vi "Lesson 3 - Exercise 3.1.2 - Cos Sin Orthogonality.vi"() -> ()   [LabVIEW 2015]
uses:
  <vilib>/Analysis/NI_AALBase.lvlib
panel:
  in  "A":dbl=3.0
  in  "B":dbl=3.0
  in  "stop":bool
  out "2*Avg( [A*Sin+B*Cos] * Sin )":dbl=2.9999999999999996 format="%.2f"
  out "1 * Sin(f)":dbl[](graph)=[0.0, 0.049067674327418015, 0.0980171403295606, 0.14673047445536175, 0.19509032201612828, 0.2429801799032639, 0.2902846772544624, 0.33688985339222005, 0.3826834323650898, 0.4275550934302821, 0.47139673682599764, 0.5141027441932218, 0.5555702330196022, 0.5956993044924334, 0.6343932841636455, 0.6715589548470184, 0.7071067811865475, 0.7409511253549591, 0.7730104533627369, 0.8032075314806449, 0.8314696123025451, 0.8577286100002721, 0.8819212643483549, 0.9039892931234433, 0.9238795325112866, 0.9415440651830208, 0.9569403357322087, 0.970031253194544, 0.9807852804032303, 0.9891765099647809, 0.9951847266721968, 0.9987954562051723, 0.9999999999999999, 0.9987954562051723, 0.9951847266721968, 0.9891765099647809, 0.9807852804032304, 0.970031253194544, 0.9569403357322088, 0.9415440651830208, 0.9238795325112867, 0.9039892931234433, 0.881921264348355, 0.8577286100002721, 0.8314696123025452, 0.8032075314806449, 0.773010453362737, 0.7409511253549591, 0.7071067811865476, 0.6715589548470184, 0.6343932841636456, 0.5956993044924334, 0.5555702330196023, 0.5141027441932218, 0.4713967368259977, 0.42755509343028214, 0.38268343236508984, 0.3368898533922201, 0.29028467725446244, 0.24298017990326393, 0.19509032201612836, 0.14673047445536178, 0.0980171403295607, 0.04906767432741803, 1.0034968732711147e-16, -0.04906767432741801, -0.0980171403295605, -0.14673047445536175, -0.19509032201612816, -0.2429801799032639, -0.2902846772544623, -0.33688985339222005, -0.38268343236508967, -0.4275550934302821, -0.47139673682599753, -0.5141027441932218, -0.5555702330196021, -0.5956993044924334, -0.6343932841636454, -0.6715589548470184, -0.7071067811865475, -0.7409511253549591, -0.7730104533627369, -0.8032075314806449, -0.8314696123025451, -0.8577286100002721, -0.8819212643483549, -0.9039892931234433, -0.9238795325112866, -0.9415440651830208, -0.9569403357322087, -0.970031253194544, -0.9807852804032303, -0.9891765099647809, -0.9951847266721968, -0.9987954562051723, -0.9999999999999999, -0.9987954562051723, -0.9951847266721968, -0.9891765099647809, -0.9807852804032304, -0.970031253194544, -0.9569403357322088, -0.9415440651830208, -0.9238795325112867, -0.9039892931234433, -0.881921264348355, -0.8577286100002721, -0.8314696123025452, -0.8032075314806449, -0.773010453362737, -0.7409511253549591, -0.7071067811865476, -0.6715589548470184, -0.6343932841636456, -0.5956993044924334, -0.5555702330196023, -0.5141027441932218, -0.4713967368259977, -0.42755509343028214, -0.38268343236508984, -0.3368898533922201, -0.29028467725446244, -0.24298017990326395, -0.19509032201612836, -0.1467304744553618, -0.0980171403295607, -0.049067674327418064]
  out "B * Cos(f)":dbl[](graph)=[3.0, 2.996386368615517, 2.9855541800165906, 2.967529529894343, 2.9423558412096913, 2.910093759583632, 2.8708210071966267, 2.824632195549062, 2.7716385975338604, 2.71196787937033, 2.6457637930450653, 2.573185830000816, 2.494408836907636, 2.4096225944419345, 2.319031360088211, 2.222853376064877, 2.121320343559643, 2.0146768645410553, 1.9031798524909367, 1.7870979134773002, 1.6667106990588068, 1.5423082325796653, 1.414190210477993, 1.2826652802908465, 1.1480502970952695, 1.0106695601766604, 0.8708540317633873, 0.728940539709792, 0.5852709660483849, 0.4401914233660856, 0.29405142098868187, 0.14720302298225438, 3.472157457384828e-17, -0.1472030229822537, -0.2940514209886818, -0.4401914233660849, -0.5852709660483848, -0.7289405397097913, -0.8708540317633872, -1.0106695601766598, -1.1480502970952693, -1.2826652802908458, -1.4141902104779929, -1.5423082325796647, -1.6667106990588065, -1.7870979134772995, -1.9031798524909365, -2.014676864541055, -2.1213203435596424, -2.2228533760648768, -2.3190313600882106, -2.409622594441934, -2.4944088369076356, -2.5731858300008157, -2.645763793045065, -2.7119678793703295, -2.77163859753386, -2.8246321955490616, -2.8708210071966263, -2.9100937595836314, -2.942355841209691, -2.9675295298943425, -2.98555418001659, -2.996386368615517, -2.9999999999999996, -2.996386368615517, -2.98555418001659, -2.967529529894343, -2.942355841209691, -2.9100937595836323, -2.8708210071966263, -2.8246321955490625, -2.77163859753386, -2.7119678793703303, -2.645763793045065, -2.5731858300008166, -2.4944088369076356, -2.409622594441935, -2.3190313600882106, -2.2228533760648777, -2.1213203435596424, -2.0146768645410558, -1.9031798524909365, -1.7870979134773006, -1.6667106990588068, -1.5423082325796658, -1.414190210477993, -1.282665280290847, -1.1480502970952695, -1.0106695601766609, -0.8708540317633874, -0.7289405397097924, -0.5852709660483851, -0.440191423366086, -0.2940514209886822, -0.1472030229822548, -4.4368263403538055e-16, 0.1472030229822533, 0.2940514209886813, 0.4401914233660845, 0.5852709660483842, 0.728940539709791, 0.8708540317633865, 1.0106695601766595, 1.1480502970952686, 1.2826652802908458, 1.4141902104779922, 1.5423082325796647, 1.6667106990588059, 1.7870979134772995, 1.9031798524909356, 2.014676864541055, 2.1213203435596415, 2.222853376064877, 2.3190313600882098, 2.409622594441935, 2.4944088369076347, 2.5731858300008166, 2.645763793045064, 2.7119678793703303, 2.771638597533859, 2.8246321955490625, 2.8708210071966254, 2.9100937595836323, 2.94235584120969, 2.9675295298943434, 2.9855541800165892, 2.996386368615518]
  out "A * Sin(f)":dbl[](graph)=[0.0, 0.14720302298225404, 0.2940514209886818, 0.44019142336608524, 0.5852709660483848, 0.7289405397097917, 0.8708540317633872, 1.0106695601766602, 1.1480502970952693, 1.2826652802908463, 1.4141902104779929, 1.542308232579665, 1.6667106990588065, 1.7870979134773, 1.9031798524909365, 2.0146768645410553, 2.1213203435596424, 2.222853376064877, 2.3190313600882106, 2.4096225944419345, 2.4944088369076356, 2.573185830000816, 2.645763793045065, 2.71196787937033, 2.77163859753386, 2.824632195549062, 2.8708210071966263, 2.910093759583632, 2.942355841209691, 2.967529529894343, 2.98555418001659, 2.996386368615517, 2.9999999999999996, 2.996386368615517, 2.98555418001659, 2.967529529894343, 2.942355841209691, 2.910093759583632, 2.8708210071966263, 2.824632195549062, 2.77163859753386, 2.71196787937033, 2.645763793045065, 2.573185830000816, 2.4944088369076356, 2.4096225944419345, 2.3190313600882106, 2.222853376064877, 2.1213203435596424, 2.0146768645410553, 1.9031798524909365, 1.7870979134773002, 1.6667106990588068, 1.5423082325796653, 1.414190210477993, 1.2826652802908465, 1.1480502970952695, 1.0106695601766604, 0.8708540317633874, 0.728940539709792, 0.5852709660483851, 0.4401914233660856, 0.29405142098868214, 0.14720302298225435, 3.703363570667362e-16, -0.14720302298225374, -0.2940514209886814, -0.44019142336608497, -0.5852709660483844, -0.7289405397097914, -0.8708540317633866, -1.01066956017666, -1.1480502970952688, -1.282665280290846, -1.4141902104779924, -1.5423082325796649, -1.666710699058806, -1.7870979134772997, -1.9031798524909358, -2.014676864541055, -2.121320343559642, -2.2228533760648768, -2.31903136008821, -2.409622594441934, -2.494408836907635, -2.5731858300008157, -2.6457637930450644, -2.7119678793703295, -2.7716385975338595, -2.8246321955490616, -2.870821007196626, -2.9100937595836314, -2.9423558412096904, -2.9675295298943425, -2.9855541800165897, -2.996386368615517, -2.999999999999999, -2.996386368615517, -2.9855541800165897, -2.967529529894343, -2.9423558412096904, -2.9100937595836323, -2.870821007196626, -2.8246321955490625, -2.7716385975338595, -2.7119678793703303, -2.6457637930450644, -2.5731858300008166, -2.494408836907635, -2.409622594441935, -2.3190313600882106, -2.2228533760648777, -2.1213203435596424, -2.0146768645410558, -1.9031798524909365, -1.7870979134773006, -1.6667106990588068, -1.5423082325796658, -1.414190210477993, -1.282665280290847, -1.1480502970952695, -1.0106695601766609, -0.8708540317633874, -0.7289405397097924, -0.5852709660483851, -0.440191423366086, -0.29405142098868225, -0.1472030229822548]
  out "A*Sin + B*Cos":dbl[](graph)=[3.0, 3.143589391597771, 3.2796056010052723, 3.4077209532604282, 3.527626807258076, 3.6390342992934235, 3.7416750389600137, 3.8353017557257223, 3.9196888946291297, 3.994633159661176, 4.059954003523059, 4.115494062580481, 4.161119535966442, 4.196720507919235, 4.222211212579148, 4.237530240605933, 4.242640687119286, 4.237530240605933, 4.222211212579147, 4.196720507919235, 4.161119535966442, 4.115494062580481, 4.059954003523058, 3.994633159661176, 3.9196888946291297, 3.8353017557257223, 3.7416750389600137, 3.639034299293424, 3.5276268072580756, 3.4077209532604287, 3.279605601005272, 3.1435893915977715, 2.9999999999999996, 2.8491833456332634, 2.6915027590279084, 2.527338106528258, 2.357084875161306, 2.1811532198738406, 1.9999669754332392, 1.8139626353724023, 1.6235883004385907, 1.429302599079484, 1.231573582567072, 1.0308775974211515, 0.8276981378488291, 0.622524680964635, 0.4158515075972742, 0.20817651152382233, 0.0, -0.20817651152382144, -0.4158515075972742, -0.6225246809646339, -0.8276981378488288, -1.0308775974211504, -1.2315735825670717, -1.429302599079483, -1.6235883004385905, -1.8139626353724012, -1.9999669754332388, -2.1811532198738393, -2.3570848751613056, -2.5273381065282567, -2.691502759027908, -2.8491833456332625, -2.999999999999999, -3.1435893915977706, -3.2796056010052714, -3.407720953260428, -3.527626807258075, -3.6390342992934235, -3.741675038960013, -3.8353017557257223, -3.919688894629129, -3.994633159661176, -4.059954003523057, -4.115494062580481, -4.161119535966442, -4.196720507919235, -4.222211212579147, -4.237530240605933, -4.242640687119284, -4.237530240605933, -4.222211212579147, -4.196720507919235, -4.161119535966442, -4.115494062580481, -4.059954003523058, -3.994633159661176, -3.919688894629129, -3.8353017557257223, -3.7416750389600133, -3.639034299293424, -3.5276268072580756, -3.4077209532604287, -3.279605601005272, -3.143589391597772, -2.9999999999999996, -2.849183345633264, -2.6915027590279084, -2.5273381065282585, -2.357084875161306, -2.181153219873841, -1.9999669754332392, -1.813962635372403, -1.623588300438591, -1.4293025990794845, -1.2315735825670722, -1.030877597421152, -0.8276981378488293, -0.6225246809646354, -0.41585150759727507, -0.20817651152382277, -8.881784197001252e-16, 0.20817651152382144, 0.4158515075972733, 0.6225246809646343, 0.827698137848828, 1.0308775974211508, 1.2315735825670708, 1.4293025990794834, 1.6235883004385896, 1.8139626353724017, 1.9999669754332379, 2.1811532198738397, 2.3570848751613047, 2.527338106528257, 2.691502759027907, 2.849183345633263]
  out "[A*Sin + B*Cos] * Sin":dbl[](graph)=[0.0, 0.15424862048604557, 0.3214575624193467, 0.5000165122833803, 0.6882058497807045, 0.8842132087164639, 1.0861509310755855, 1.2920742462013628, 1.5, 1.7079257537986372, 1.9138490689244148, 2.115786791283536, 2.311794150219295, 2.49998348771662, 2.6785424375806537, 2.845751379513955, 3.0, 3.1398028005026366, 3.263813403629037, 3.370837519480007, 3.459844447314564, 3.5299770017615293, 3.5805597679832206, 3.6111056062895734, 3.6213203435596424, 3.6111056062895734, 3.5805597679832206, 3.5299770017615293, 3.459844447314564, 3.3708375194800073, 3.263813403629037, 3.139802800502636, 2.999999999999999, 2.8457513795139544, 2.678542437580653, 2.49998348771662, 2.311794150219295, 2.1157867912835364, 1.913849068924414, 1.7079257537986374, 1.4999999999999998, 1.2920742462013632, 1.0861509310755852, 0.8842132087164644, 0.6882058497807045, 0.5000165122833805, 0.3214575624193466, 0.15424862048604576, 0.0, -0.13980280050263583, -0.263813403629038, -0.3708375194800064, -0.45984444731456475, -0.5299770017615287, -0.5805597679832211, -0.6111056062895734, -0.6213203435596425, -0.6111056062895734, -0.5805597679832212, -0.5299770017615288, -0.4598444473145648, -0.37083751948000676, -0.26381340362903827, -0.13980280050263624, -3.010490619813343e-16, 0.1542486204860455, 0.3214575624193463, 0.5000165122833802, 0.688205849780704, 0.8842132087164639, 1.0861509310755848, 1.2920742462013628, 1.4999999999999993, 1.7079257537986372, 1.9138490689244134, 2.115786791283536, 2.3117941502192947, 2.49998348771662, 2.6785424375806524, 2.845751379513955, 2.9999999999999987, 3.1398028005026366, 3.263813403629037, 3.370837519480007, 3.459844447314564, 3.5299770017615293, 3.5805597679832206, 3.6111056062895734, 3.6213203435596415, 3.6111056062895734, 3.58055976798322, 3.5299770017615293, 3.459844447314564, 3.3708375194800073, 3.263813403629037, 3.1398028005026366, 2.999999999999999, 2.845751379513955, 2.678542437580653, 2.4999834877166203, 2.311794150219295, 2.115786791283537, 1.913849068924414, 1.707925753798638, 1.5, 1.2920742462013635, 1.0861509310755855, 0.8842132087164647, 0.6882058497807048, 0.5000165122833808, 0.32145756241934725, 0.1542486204860461, 6.280369834735101e-16, -0.13980280050263583, -0.26381340362903744, -0.37083751948000665, -0.45984444731456425, -0.529977001761529, -0.5805597679832206, -0.6111056062895737, -0.6213203435596422, -0.6111056062895737, -0.5805597679832208, -0.5299770017615291, -0.45984444731456464, -0.3708375194800069, -0.26381340362903816, -0.13980280050263635]
  # "*Set A to zero: BCos (*) Sin = 0\n   -for all B -> Cos:Sin orthogonal\n*Set A to non-zero\n   - any change in B does not effect our ability to calculate A! \n\nTakeaway:\nWe can always calculate out A, regardless of what B is.\n\nFor explanation of math, see block diagram"
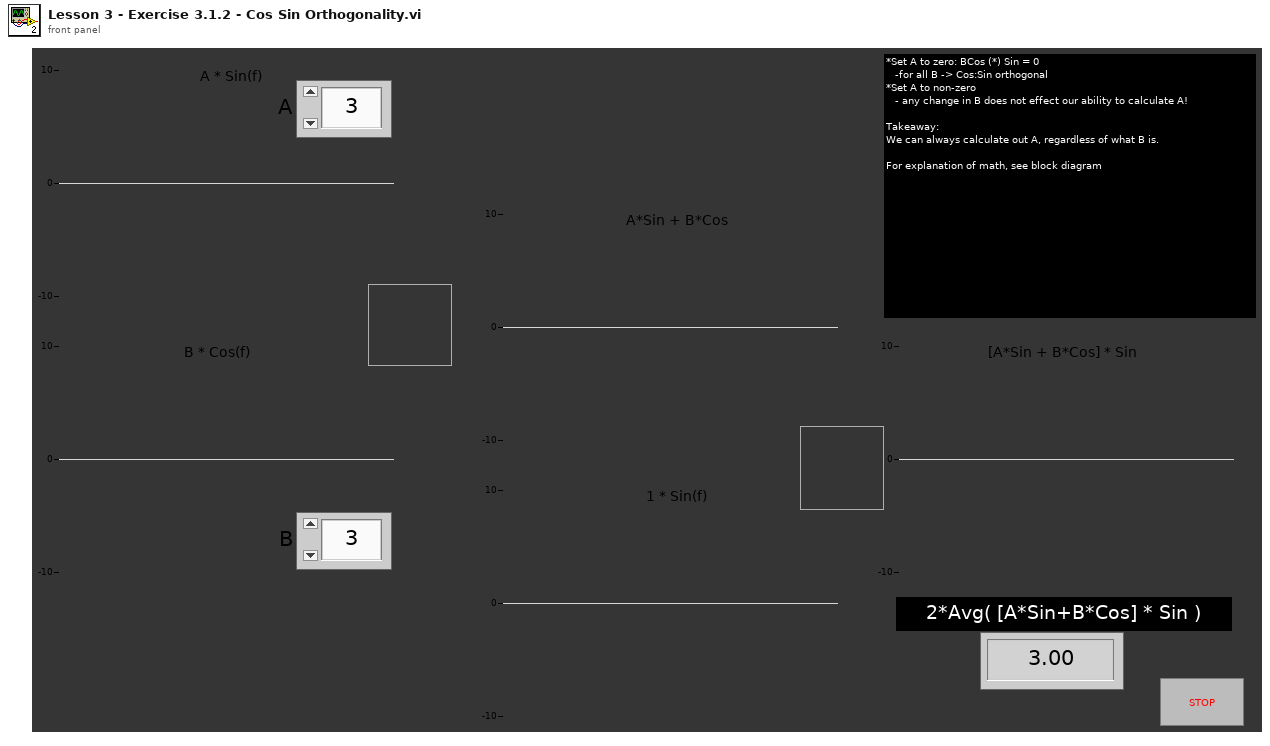
[diagram p1: front panel]
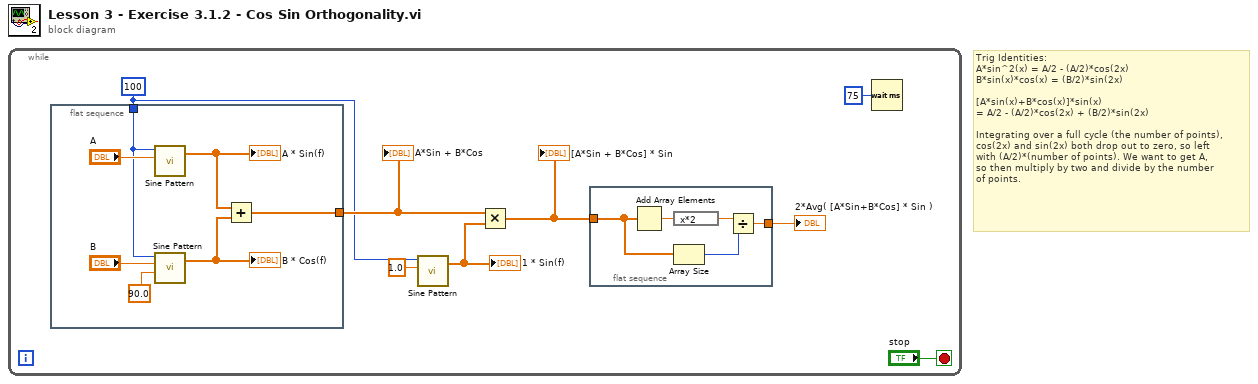
[diagram p0: block diagram]
diagram:
  # "Trig Identities:\nA*sin^2(x) = A/2 - (A/2)*cos(2x)\nB*sin(x)*cos(x) = (B/2)*sin(2x)\n\n[A*sin(x)+B*cos(x)]*sin(x) \n= A/2 - (A/2)*cos(2x) + (B/2)*sin(2x) \n\nIntegrating over a full cycle (the number of points), \ncos(2x) and sin(2x) both drop out to zero, so left \nwith (A/2)*(number of points). We want to get A, \nso then multiply by two and divide by the number\nof points."
  n1 = while {
    stop <- "stop" stop-if-true
    w1 = 100 ("samples")
    n2 = flat-sequence {
      tunnel: [w16] -> w7
      tunnel: w1 -> [w14]
      frame #0 {
        n3 = call <vilib>:"Sine Pattern.vi"("amplitude"="A", "samples"=w14) -> ("Sinusoidal Pattern"=w18:dbl[])  [unwired: 2 in, 1 out]
        "A * Sin(f)" <- w18
        n4 = call <vilib>:"Sine Pattern.vi"("phase(degrees)"=90.0, "amplitude"="B", "samples"=w14) -> ("Sinusoidal Pattern"=w17:dbl[])  [unwired: 1 in, 1 out]
        "B * Cos(f)" <- w17
        n5 = Add(x=w18, y=w17) -> (x+y=w16:dbl[])
      }
    }
    n6 = call <vilib>:"Sine Pattern.vi"("amplitude"=1.0, "samples"=w1) -> ("Sinusoidal Pattern"=w6:dbl[])  [unwired: 2 in, 1 out]
    "1 * Sin(f)" <- w6
    n7 = Multiply(x=w7, y=w6) -> (x*y=w4:dbl[])
    "[A*Sin + B*Cos] * Sin" <- w4
    n8 = flat-sequence "Cosine integrates to zero, only left w/ 1/2 * A\nZ*Sin^2(x) = 1/2*Z - 1/2 cos(2x)" {
      tunnel: [w10] -> w5
      tunnel: w4 -> [w9]
      frame #0 {
        n9 = Add Array Elements(numeric array=w9) -> (sum=w11:dbl)
        n10 = expression code="x*2"(w11) -> (w12:dbl)
        n11 = Array Size(array=w9) -> (size(s)=w13:i32)
        n12 = Divide(x=w12, y=w13) -> (x/y=w10:dbl)
      }
    }
    n13 = Wait (ms)(milliseconds to wait=u32 75) -> ()  [unwired: 1 out]
    "A*Sin + B*Cos" <- w7
    "2*Avg( [A*Sin+B*Cos] * Sin )" <- w5
  }
